vi "VoltFilter.vi"(8 "error in (no error)":errorcluster, 11 "Voltage In [V]":dbl) -> (0 "error out":errorcluster, 3 "Voltage Out [V]":dbl)   [LabVIEW 2018, in "WeightMeas.lvlib"]
doc: "Voltage filtering, to get a more averaged value."
uses:
  WeightMeas.lvlib
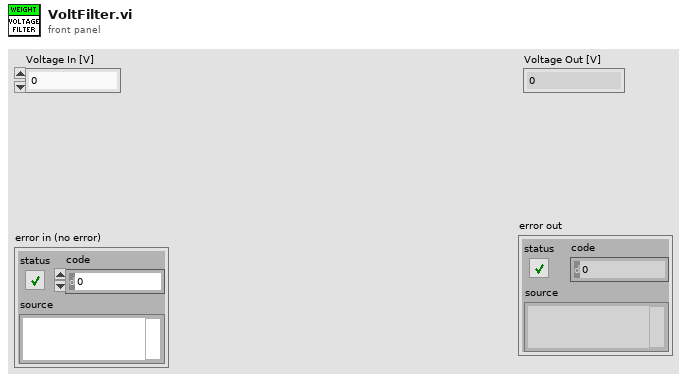
[diagram p1: front panel]
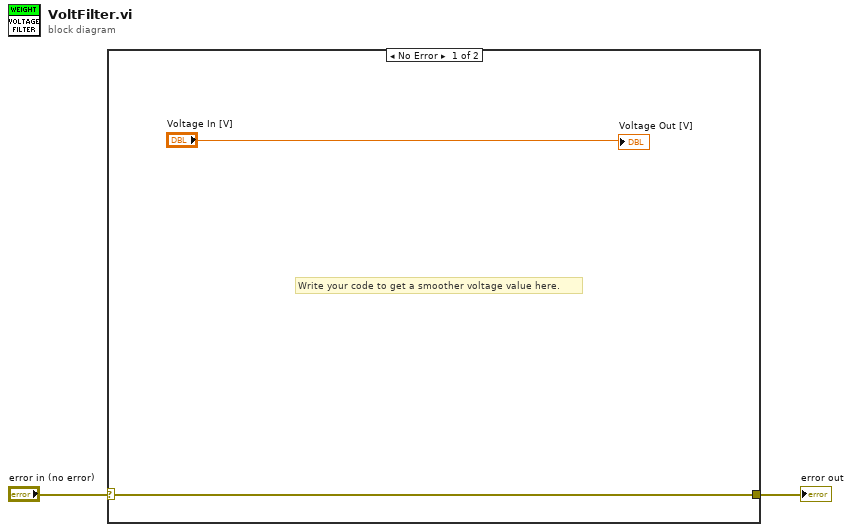
[diagram p0: block diagram]
diagram:
  n1 = case shown="No Error" "error in (no error)" {
    selector: "error in (no error)" -> [w4 w5]
    tunnel: [w4 w5] -> w1
    frame No Error {
      # "Write your code to get a smoother voltage value here."
      "Voltage Out [V]" <- "Voltage In [V]"
    }
    frame Error {
      # "Leave empty, this case is for error handling."
    }
  }
  "error out" <- w1
